vi "ShooterControl.vi"(0 "ShooterTop":T1={"DeviceStatus"={"status"=FALSE, "code"=0, "source"=""}, "Type"=enum."PWM", "PWM"={"Digital Module"=enum."Digital Module 1", "PWM Channel"=enum."Invalid", "DeadBand"={"Name"="", "maxPositivePwm"=0, "minPositivePwm"=0, "centerPwm"=0, "maxNegativePwm"=0, "minNegativePwm"=0, "angularRange"=0}}, "CAN"={"Device Number"=0, "Control Mode"=enum."Percent VBus", "Semaphore"=refnum, "Max Vout"=12.0}, "Invert"=FALSE, "TransformRef"=refnum, "InvTransformRef"=refnum}, 1 "ShooterBottom":T1={"DeviceStatus"={"status"=FALSE, "code"=0, "source"=""}, "Type"=enum."PWM", "PWM"={"Digital Module"=enum."Digital Module 1", "PWM Channel"=enum."Invalid", "DeadBand"={"Name"="", "maxPositivePwm"=0, "minPositivePwm"=0, "centerPwm"=0, "maxNegativePwm"=0, "minNegativePwm"=0, "angularRange"=0}}, "CAN"={"Device Number"=0, "Control Mode"=enum."Percent VBus", "Semaphore"=refnum, "Max Vout"=12.0}, "Invert"=FALSE, "TransformRef"=refnum, "InvTransformRef"=refnum}, 2 "ThrottleAxis":dbl, 3 "AutoTrack":bool, 4 "ClosedLoopKillSwitch":bool, 5 "ON/OFF":bool, 6 "TopEnc":dbl, 7 "OpenLoopMax":dbl, 8 "BotEnc":dbl, 9 "OpenLoopMin":dbl, 10 "button6":bool, 11 "ClosedLoopMax":dbl, 12 "Distance":dbl, 13 "ClosedLoopMin":dbl, 18 "button8":bool, 19 "button7":bool) -> (14 "ShooterTop":T1={"DeviceStatus"={"status"=FALSE, "code"=0, "source"=""}, "Type"=enum."PWM", "PWM"={"Digital Module"=enum."Digital Module 1", "PWM Channel"=enum."Invalid", "DeadBand"={"Name"="", "maxPositivePwm"=0, "minPositivePwm"=0, "centerPwm"=0, "maxNegativePwm"=0, "minNegativePwm"=0, "angularRange"=0}}, "CAN"={"Device Number"=0, "Control Mode"=enum."Percent VBus", "Semaphore"=refnum, "Max Vout"=12.0}, "Invert"=FALSE, "TransformRef"=refnum, "InvTransformRef"=refnum}, 15 "ShooterTopValue":dbl, 16 "ShooterBottom":T1={"DeviceStatus"={"status"=FALSE, "code"=0, "source"=""}, "Type"=enum."PWM", "PWM"={"Digital Module"=enum."Digital Module 1", "PWM Channel"=enum."Invalid", "DeadBand"={"Name"="", "maxPositivePwm"=0, "minPositivePwm"=0, "centerPwm"=0, "maxNegativePwm"=0, "minNegativePwm"=0, "angularRange"=0}}, "CAN"={"Device Number"=0, "Control Mode"=enum."Percent VBus", "Semaphore"=refnum, "Max Vout"=12.0}, "Invert"=FALSE, "TransformRef"=refnum, "InvTransformRef"=refnum}, 17 "ShooterBottomValue":dbl)   [LabVIEW 2011]
uses:
  <vilib>/Rock Robotics/WPI/MotorControl/WPI_MotorControlDeviceRef.ctl
  <vilib>/Rock Robotics/SystemInterfaces/Typedef/FPGA_TypedefDigitalModule.ctl
  <vilib>/Rock Robotics/SystemInterfaces/DIO/FPGA_DIOPWMChannel.ctl
  <vilib>/Rock Robotics/WPI/PWM/WPI_PWMDeadband.ctl
  <vilib>/Rock Robotics/WPI/CAN/Jaguar/SubVIs/WPI_CANJaguar_ControlMode.ctl
  <vilib>/Rock Robotics/WPI/PWM/WPI_PWMTransform_ConPane.ctl
  <vilib>/Rock Robotics/WPI/DriverStation/DriverStationLCD/WPI_DriverStationLCDLCDLine.ctl
  <vilib>/Rock Robotics/WPI/CAN/Jaguar/SubVIs/WPI_CANJaguar_SpeedReference.ctl
  Robot Global Data.vi
panel:
  in  "Add Num":dbl
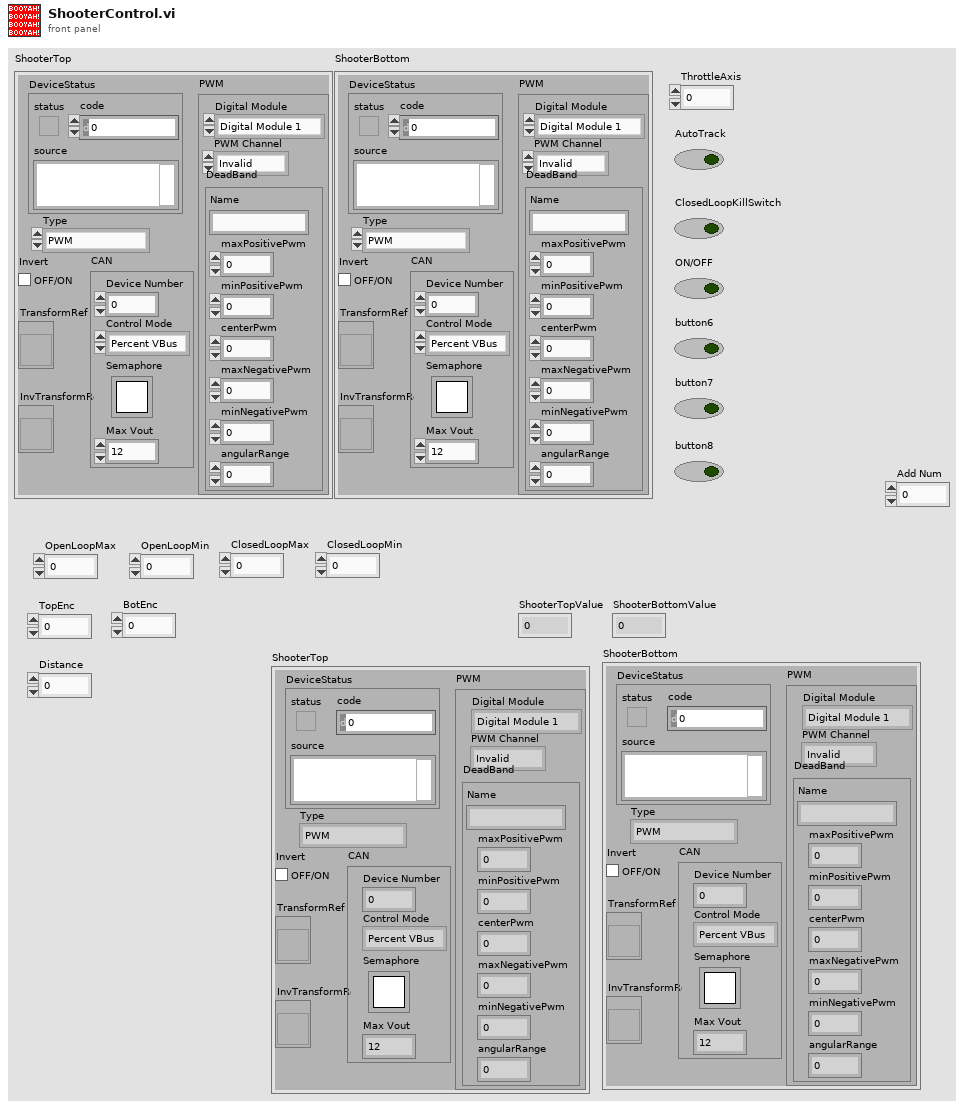
[diagram p1: front panel]
types:
  T1 = typedef "WPI_MotorControlDeviceRef.ctl" = cluster{"DeviceStatus":errorcluster, "Type":enum16{"PWM", "CAN"}, "PWM":cluster{"Digital Module":T2, "PWM Channel":T3, "DeadBand":T4}, "CAN":cluster{"Device Number":u8, "Control Mode":T5, "Semaphore":T6, "Max Vout":dbl}, "Invert":bool, "TransformRef":T7, "InvTransformRef":T7}
  T2 = typedef "FPGA_TypedefDigitalModule.ctl" = enum16{"Digital Module 1", "Digital Module 2"}
  T3 = typedef "FPGA_DIOPWMChannel.ctl" = enum8{"PWM 1", "PWM 2", "PWM 3", "PWM 4", "PWM 5", "PWM 6", "PWM 7", "PWM 8", "PWM 9", "PWM 10", "Invalid"}
  T4 = typedef "WPI_PWMDeadband.ctl" = cluster{"Name":string, "maxPositivePwm":i32, "minPositivePwm":i32, "centerPwm":i32, "maxNegativePwm":i32, "minNegativePwm":i32, "angularRange":u16}
  T5 = typedef "WPI_CANJaguar_ControlMode.ctl" = enum8{"Percent VBus", "Current", "Speed", "Position", "Voltage"}
  T6 = typedef "Semaphore RefNum" = refnum<k1>
  T7 = typedef "WPI_PWMTransform_ConPane.ctl" = refnum<vi>
  T8 = typedef "WPI_DriverStationLCDLCDLine.ctl" = enum16{"Main - Line 1", "User - Line 2", "User - Line 3", "User - Line 4", "User - Line 5", "User - Line 6"}
  T9 = typedef "WPI_CANJaguar_SpeedReference.ctl" = u8
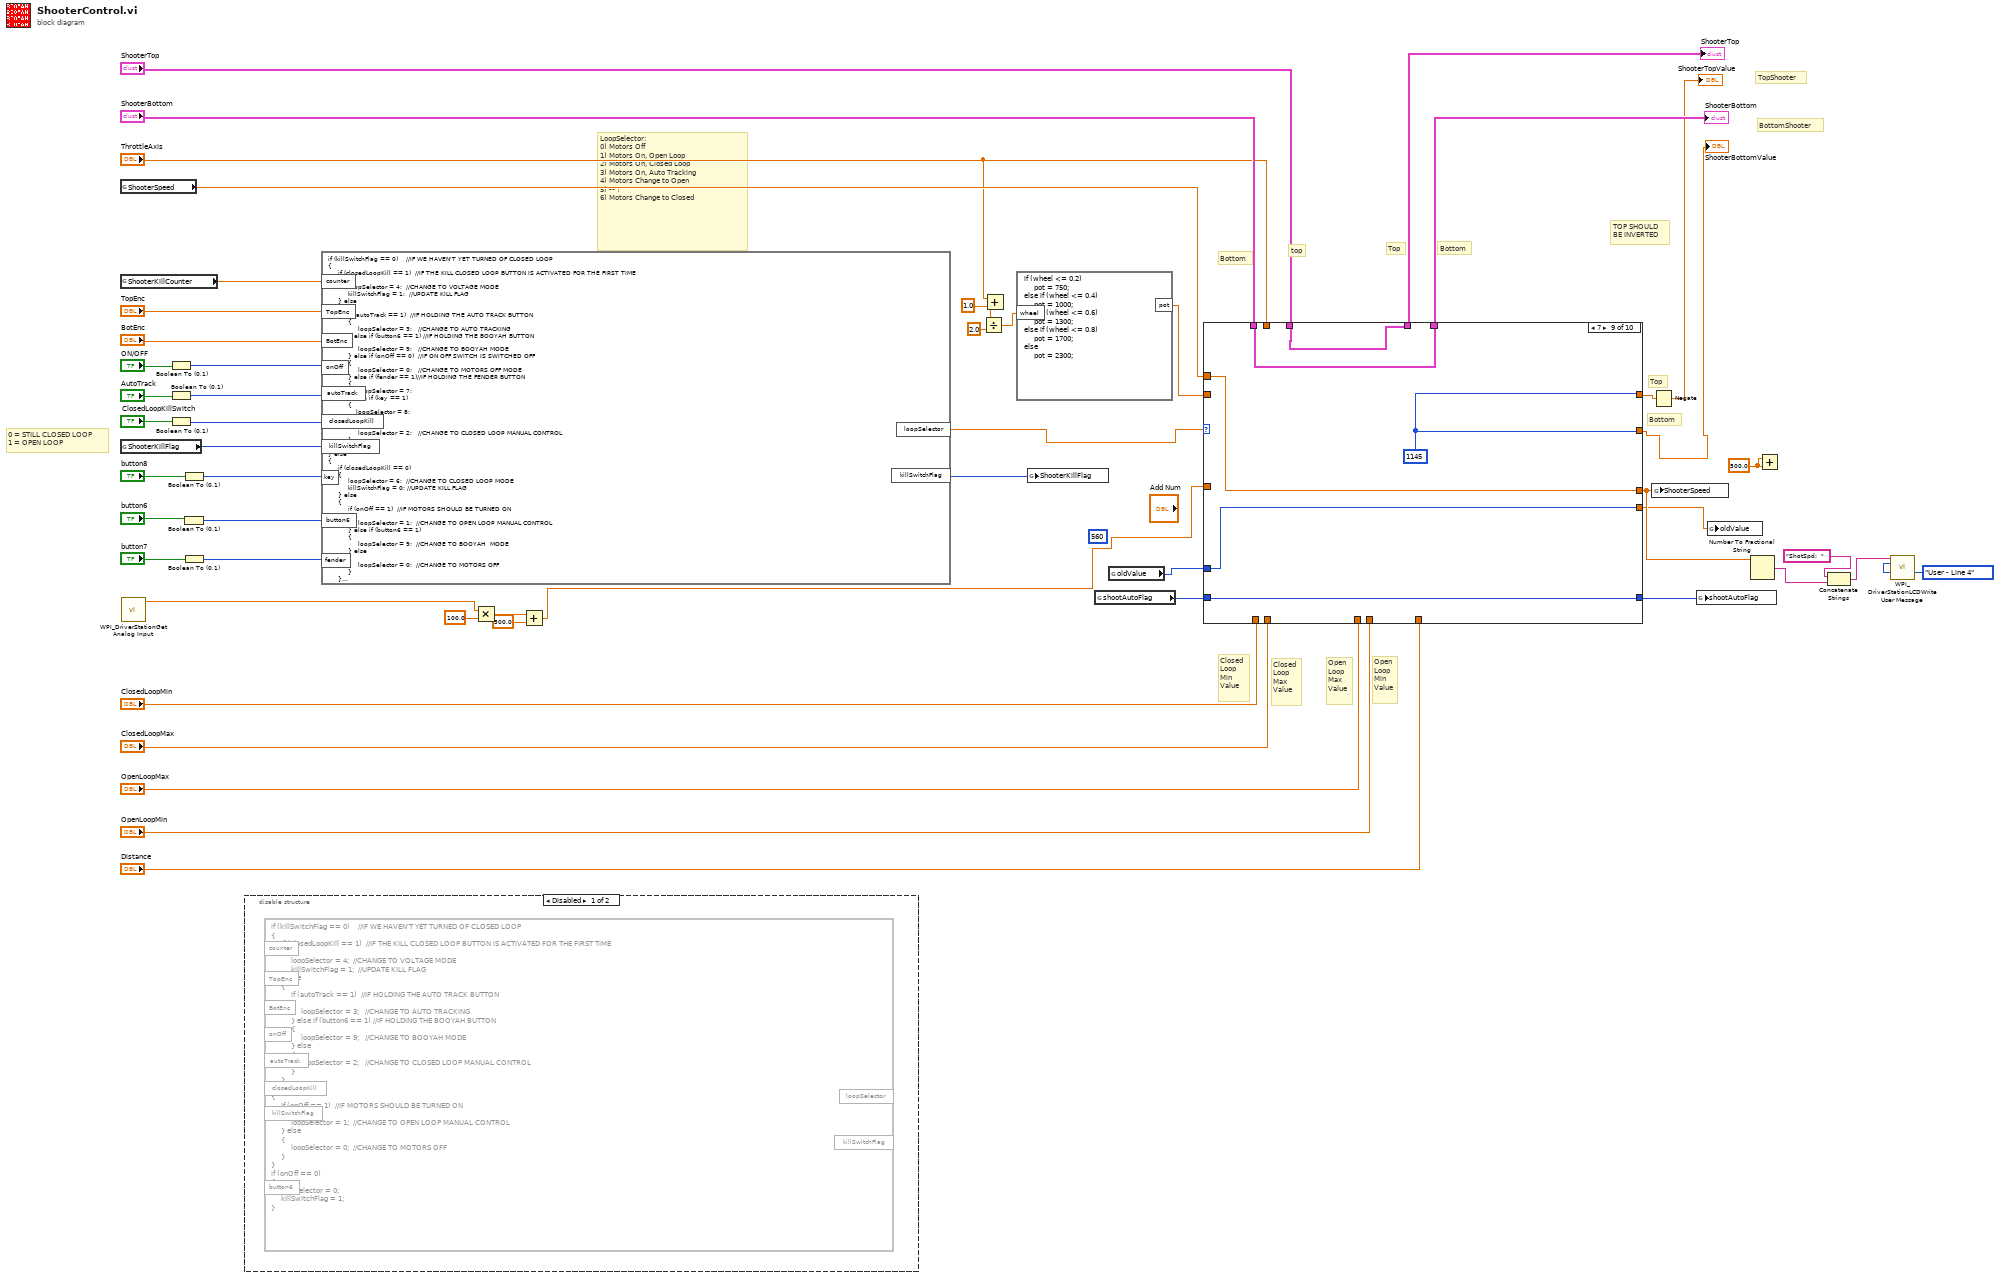
[diagram p0: block diagram]
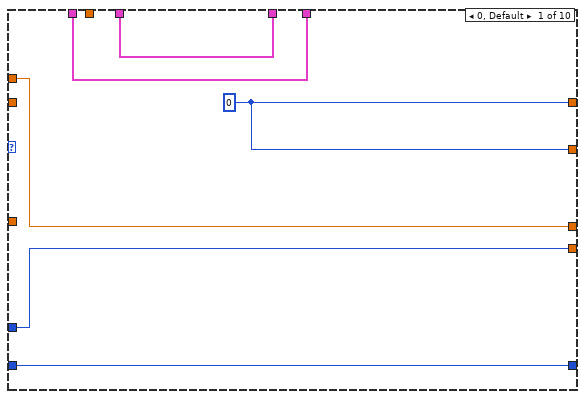
[diagram p3: hidden frame]
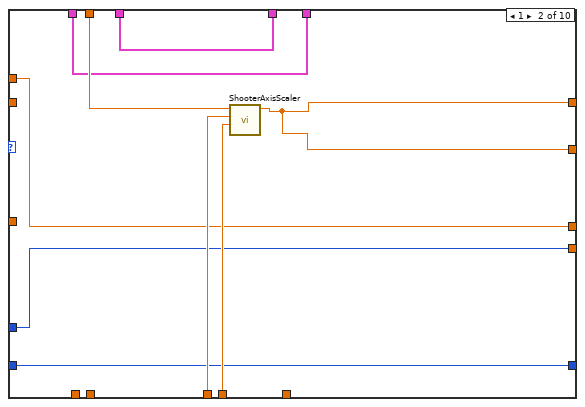
[diagram p4: hidden frame]
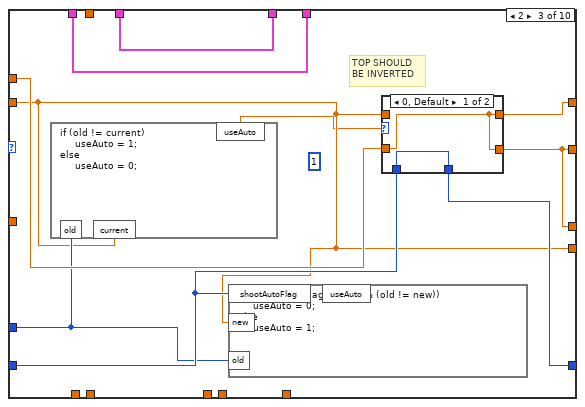
[diagram p5: hidden frame]
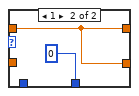
[diagram p6: hidden frame]
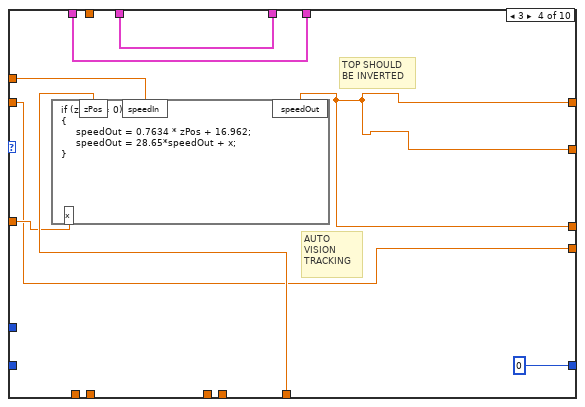
[diagram p7: hidden frame]
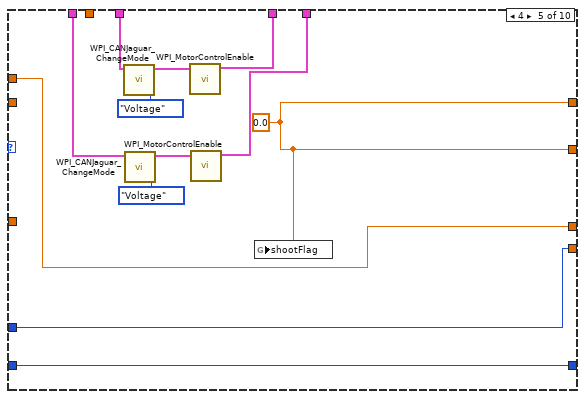
[diagram p8: hidden frame]
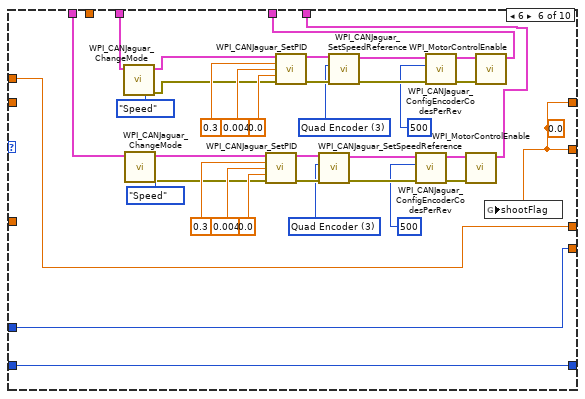
[diagram p9: hidden frame]
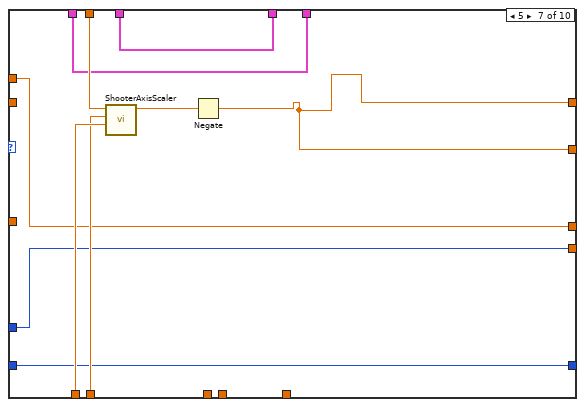
[diagram p10: hidden frame]
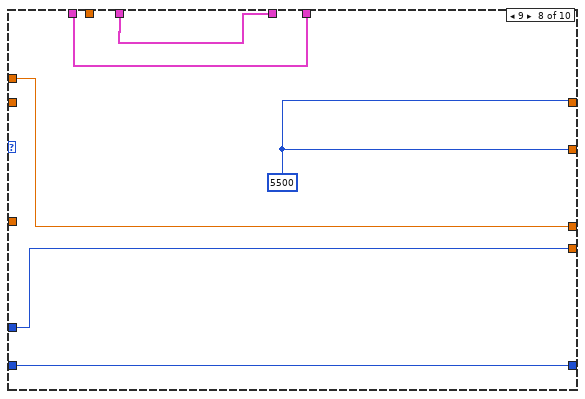
[diagram p11: hidden frame]
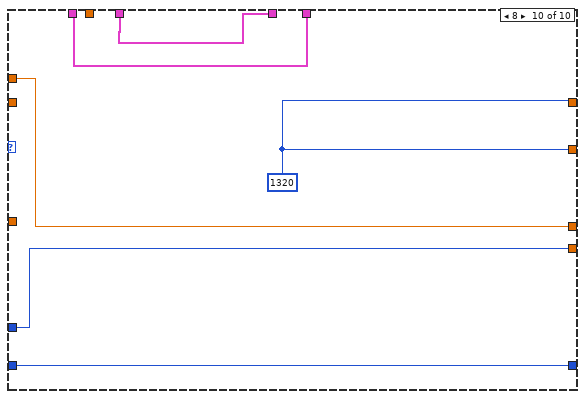
[diagram p12: hidden frame]
diagram:
  (unwired) 560
  w26 = 500.0 ("y")
  # "TOP SHOULD\nBE INVERTED"
  # "0 = STILL CLOSED LOOP\n1 = OPEN LOOP"
  # "Bottom"
  # "Top"
  # "top"
  # "Bottom"
  # "Closed\nLoop\nMin\nValue"
  # "Closed\nLoop\nMax\nValue"
  # "Open\nLoop\nMax\nValue"
  # "Open\nLoop\nMin\nValue"
  # "Bottom"
  # "BottomShooter"
  # "TopShooter"
  # "Top"
  # "LoopSelector:\n0) Motors Off\n1) Motors On, Open Loop\n2) Motors On, Closed Loop\n3) Motors On, Auto Tracking\n4) Motors Change to Open\n5) -- ?\n6) Motors Change to Closed"
  n1 = global read "Robot Global Data.vi" "ShooterSpeed"() -> (w29:dbl)
  n2 = global read "Robot Global Data.vi" "ShooterKillCounter"() -> (w33:dbl)
  n3 = global read "Robot Global Data.vi" "ShooterKillFlag"() -> (w38:u8)
  n4 = call <vilib>:"WPI_DriverStationGet Analog Input.vi"() -> ("Analog 1 (V)"=w23:dbl)  [unwired: 8 in, 3 out]
  n5 = Boolean To (0,1)(Boolean="ON/OFF") -> (0, 1=w47:i16)
  n6 = Boolean To (0,1)(Boolean="AutoTrack") -> (0, 1=w49:i16)
  n7 = Boolean To (0,1)(Boolean="ClosedLoopKillSwitch") -> (0, 1=w51:i16)
  n8 = Boolean To (0,1)(Boolean="button6") -> (0, 1=w31:i16)
  n9 = Boolean To (0,1)(Boolean="button8") -> (0, 1=w2:i16)
  n10 = Boolean To (0,1)(Boolean="button7") -> (0, 1=w24:i16)
  n11 = disable-structure shown="Disabled" {
    frame Disabled {
      n12 = formula code="if (killSwitchFlag == 0)    //IF WE HAVEN'T YET TURNED OF CLOSED LOOP\n{\n     if (closedLoopKill == 1)  //IF THE KILL CLOSED LOOP BUTTON IS ACTIVATED FOR THE FIRST TIME\n     {\n          loopSelector = 4;  //CHANGE TO VOLTAGE MODE\n          killSwitchFlag = 1;  //UPDATE KILL FLAG\n     } else\n     {\n          if (autoTrack == 1)  //IF HOLDING THE AUTO TRACK BUTTON\n          {\n               loopSelector = 3;   //CHANGE TO AUTO TRACKING\n          } else if (button6 == 1) //IF HOLDING THE BOOYAH BUTTON\n          {\n               loopSelector = 9;   //CHANGE TO BOOYAH MODE\n          } else\n          {\n               loopSelector = 2;   //CHANGE TO CLOSED LOOP MANUAL CONTROL\n          }\n     }\n} else\n{\n     if (onOff == 1)  //IF MOTORS SHOULD BE TURNED ON\n     {\n          loopSelector = 1;  //CHANGE TO OPEN LOOP MANUAL CONTROL\n     } else\n     {\n          loopSelector = 0;  //CHANGE TO MOTORS OFF\n     }\n}\nif (onOff == 0)\n{\n     loopSelector = 0;\n     killSwitchFlag = 1;\n}"() -> ()  [unwired: 8 in, 2 out]
    }
    frame Enabled {
    }
  }
  n13 = formula code="if (killSwitchFlag == 0)    //IF WE HAVEN'T YET TURNED OF CLOSED LOOP\n{\n     if (closedLoopKill == 1)  //IF THE KILL CLOSED LOOP BUTTON IS ACTIVATED FOR THE FIRST TIME\n     {\n          loopSelector = 4;  //CHANGE TO VOLTAGE MODE\n          killSwitchFlag = 1;  //UPDATE KILL FLAG\n     } else\n     {\n          if (autoTrack == 1)  //IF HOLDING THE AUTO TRACK BUTTON\n          {\n               loopSelector = 3;   //CHANGE TO AUTO TRACKING\n          } else if (button6 == 1) //IF HOLDING THE BOOYAH BUTTON\n          {\n               loopSelector = 9;   //CHANGE TO BOOYAH MODE\n          } else if (onOff == 0)  //IF ON OFF SWITCH IS SWITCHED OFF\n          {\n               loopSelector = 0;   //CHANGE TO MOTORS OFF MODE\n          } else if (fender == 1)//IF HOLDING THE FENDER BUTTON\n          {\n               loopSelector = 7;\n          } else if (key == 1)\n          {\n              loopSelector = 8;\n          } else \n          {\n               loopSelector = 2;   //CHANGE TO CLOSED LOOP MANUAL CONTROL\n          }\n     }\n} else\n{\n     if (closedLoopKill == 0)\n     {\n          loopSelector = 6;  //CHANGE TO CLOSED LOOP MODE\n          killSwitchFlag = 0; //UPDATE KILL FLAG\n     } else\n     {\n          if (onOff == 1)  //IF MOTORS SHOULD BE TURNED ON\n          {\n               loopSelector = 1;  //CHANGE TO OPEN LOOP MANUAL CONTROL\n          } else if (button6 == 1)\n          {\n               loopSelector = 9;  //CHANGE TO BOOYAH  MODE\n          } else          \n          {\n               loopSelector = 0;  //CHANGE TO MOTORS OFF\n          }\n     }\n}"("onOff"=w47, "autoTrack"=w49, "closedLoopKill"=w51, "killSwitchFlag"=w38, "TopEnc"="TopEnc", "BotEnc"="BotEnc", "counter"=w33, "button6"=w31, "fender"=w24, "key"=w2) -> ("loopSelector"=w36:dbl, "killSwitchFlag"=w37:u8)
  n14 = Multiply(x=w23, y=100.0) -> (x*y=w21:dbl)
  n15 = Add(x=w21, y=500.0) -> (x+y=w19:dbl)
  n16 = Add(x="ThrottleAxis", y=1.0) -> (x+y=w9:dbl)
  n17 = Divide(x=w9, y=2.0) -> (x/y=w11:dbl)
  n18 = formula code="if (wheel <= 0.2)\n     pot = 750;\nelse if (wheel <= 0.4)\n     pot = 1000;\nelse if (wheel <= 0.6)\n     pot = 1300;\nelse if (wheel <= 0.8)\n     pot = 1700;\nelse\n     pot = 2300;"("wheel"=w11) -> ("pot"=w6:dbl)
  n19 = global write "Robot Global Data.vi" "ShooterKillFlag"(w37) -> ()
  n20 = global read "Robot Global Data.vi" "shootAutoFlag"() -> (w27:i8)
  n21 = global read "Robot Global Data.vi" "oldValue"() -> (w12:i32)
  n22 = case shown="7" w36 {
    tunnel: [w58 w60 w75 w84 w93 w133 w139 w149 w155 w161] -> w3
    tunnel: [w58 w60 w71 w84 w93 w133 w139 w149 w155 w161] -> w5
    tunnel: "OpenLoopMax" -> [_ w67 _ _ _ _ _ _ _ _]
    tunnel: "OpenLoopMin" -> [_ w66 _ _ _ _ _ _ _ _]
    tunnel: "ThrottleAxis" -> [_ w65 _ _ _ _ w147 _ _ _]
    tunnel: "ClosedLoopMin" -> [_ _ _ _ _ _ w146 _ _ _]
    tunnel: "ClosedLoopMax" -> [_ _ _ _ _ _ w145 _ _ _]
    tunnel: "ShooterTop" -> [w57 w64 w77 w89 w97 w135 w144 w153 w159 w165]
    tunnel: "ShooterBottom" -> [w56 w63 w76 w88 w96 w134 w143 w152 w158 w164]
    tunnel: [w57 w64 w77 w89 w95 w105 w144 w153 w159 w165] -> w40
    tunnel: [w56 w63 w76 w88 w94 w104 w143 w152 w158 w164] -> w39
    tunnel: "Distance" -> [_ _ _ w87 _ _ _ _ _ _]
    tunnel: [w55 w62 w71 w84 w92 w132 w141 w151 w157 w163] -> w14
    tunnel: w29 -> [w55 w62 w72 w86 w92 w132 w141 w151 w157 w163]
    tunnel: [w54 w61 w74 0 w91 w103 w140 w150 w156 w162] -> w28
    tunnel: w27 -> [w54 w61 w73 _ w91 w103 w140 w150 w156 w162]
    tunnel: [w53 w59 w69 w82 w90 w102 w138 w148 w154 w160] -> w13
    tunnel: w12 -> [w53 w59 w70 _ w90 w102 w138 w148 w154 w160]
    tunnel: w19 -> [_ _ _ w83 _ _ _ _ _ _]
    tunnel: w6 -> [_ _ w69 w82 _ _ _ _ _ _]
    frame 0, Default {
      w58 = 0
    }
    frame 1 {
      n23 = call "ShooterAxisScaler.vi"("MinValue"=w66, "MaxValue"=w67, "ThrottleAxisIn"=w65) -> ("ScaledThrottleOut"=w60:dbl)  [unwired: 8 in]
    }
    frame 2 {
      (unwired) 1
      # "TOP SHOULD\nBE INVERTED"
      n24 = formula code="if (old != current)\n     useAuto = 1;\nelse\n     useAuto = 0;"("old"=w70, "current"=w69) -> ("useAuto"=w68:dbl)
      n25 = formula code="if ((shootAutoFlag == 1) && (old != new))\n     useAuto = 0;\nelse\n     useAuto = 1;"("shootAutoFlag"=w73, "old"=w70, "new"=w69) -> ()  [unwired: 1 out]
      n26 = case shown="0, Default" w68 {
        tunnel: [w78 w81] -> w75
        tunnel: w69 -> [_ w81]
        tunnel: [w78 w81] -> w71
        tunnel: [w79 0] -> w74
        tunnel: w73 -> [w79 _]
        tunnel: w72 -> [w78 _]
        frame 0, Default {
        }
        frame 1 {
        }
      }
    }
    frame 3 {
      # "TOP SHOULD\nBE INVERTED"
      # "AUTO\nVISION\nTRACKING"
      n27 = formula code="if (zPos != 0)\n{\n     speedOut = 0.7634 * zPos + 16.962;\n     speedOut = 28.65*speedOut + x;\n}"("zPos"=w87, "speedIn"=w86, "x"=w83) -> ("speedOut"=w84:dbl)
    }
    frame 4 {
      w93 = 0.0 ("ScaledThrottleOut")
      n28 = call <vilib>:"WPI_CANJaguar_ChangeMode.vi"("Control Mode"=WPI_CANJaguar_ControlMode."Voltage", "CAN Jaguar Ref"=w97) -> ("CAN Jaguar Ref Out"=w100:T1)  [unwired: 1 in, 8 out]
      n29 = call <vilib>:"WPI_CANJaguar_ChangeMode.vi"("Control Mode"=WPI_CANJaguar_ControlMode."Voltage", "CAN Jaguar Ref"=w96) -> ("CAN Jaguar Ref Out"=w98:T1)  [unwired: 1 in, 8 out]
      n30 = call <vilib>:"WPI_MotorControlEnable.vi"("CAN Jaguar Ref"=w100) -> ("CAN Jaguar Ref Out"=w95:T1)  [unwired: 2 in, 8 out]
      n31 = call <vilib>:"WPI_MotorControlEnable.vi"("CAN Jaguar Ref"=w98) -> ("CAN Jaguar Ref Out"=w94:T1)  [unwired: 2 in, 8 out]
      n32 = global write "Robot Global Data.vi" "shootFlag"(w93) -> ()
    }
    frame 6 {
      w113 = T9 3 items=["Encoder"=0, "Inv Encoder"=2, "Quad Encoder"=3, "None"=255] ("Speed Reference")
      w126 = T9 3 items=["Encoder"=0, "Inv Encoder"=2, "Quad Encoder"=3, "None"=255] ("Speed Reference")
      w133 = 0.0 ("ScaledThrottleOut")
      n33 = call <vilib>:"WPI_CANJaguar_ChangeMode.vi"("Control Mode"=WPI_CANJaguar_ControlMode."Speed", "CAN Jaguar Ref"=w135) -> ("error out"=w119:errorcluster, "CAN Jaguar Ref Out"=w120:T1)  [unwired: 1 in, 7 out]
      n34 = call <vilib>:"WPI_CANJaguar_ChangeMode.vi"("Control Mode"=WPI_CANJaguar_ControlMode."Speed", "CAN Jaguar Ref"=w134) -> ("error out"=w106:errorcluster, "CAN Jaguar Ref Out"=w107:T1)  [unwired: 1 in, 7 out]
      n35 = call <vilib>:"WPI_CANJaguar_SetPID.vi"("CAN Jaguar Ref"=w107, "P"=0.3, "I"=0.004, "D"=0.0, "error in (no error)"=w106) -> ("CAN Jaguar Ref Out"=w114:T1, "error out"=w115:errorcluster)  [unwired: 9 in]
      n36 = call <vilib>:"WPI_CANJaguar_SetPID.vi"("CAN Jaguar Ref"=w120, "P"=0.3, "I"=0.004, "D"=0.0, "error in (no error)"=w119) -> ("CAN Jaguar Ref Out"=w127:T1, "error out"=w128:errorcluster)  [unwired: 9 in]
      n37 = call <vilib>:"WPI_CANJaguar_SetSpeedReference.vi"("error in (no error)"=w115, "Speed Reference"=w113, "CAN Jaguar Ref"=w114) -> ("error out"=w112:errorcluster, "CAN Jaguar Ref Out"=w111:T1)  [unwired: 7 in]
      n38 = call <vilib>:"WPI_CANJaguar_SetSpeedReference.vi"("error in (no error)"=w128, "Speed Reference"=w126, "CAN Jaguar Ref"=w127) -> ("error out"=w125:errorcluster, "CAN Jaguar Ref Out"=w124:T1)  [unwired: 7 in]
      n39 = call <vilib>:"WPI_CANJaguar_ConfigEncoderCodesPerRev.vi"("error in (no error)"=w112, "Encoder Codes Per Rev"=u16 500, "CAN Jaguar Ref"=w111) -> ("error out"=w108:errorcluster, "CAN Jaguar Ref Out"=w109:T1)  [unwired: 7 in]
      n40 = call <vilib>:"WPI_CANJaguar_ConfigEncoderCodesPerRev.vi"("error in (no error)"=w125, "Encoder Codes Per Rev"=u16 500, "CAN Jaguar Ref"=w124) -> ("error out"=w121:errorcluster, "CAN Jaguar Ref Out"=w122:T1)  [unwired: 7 in]
      n41 = call <vilib>:"WPI_MotorControlEnable.vi"("error in (no error)"=w108, "CAN Jaguar Ref"=w109) -> ("CAN Jaguar Ref Out"=w104:T1)  [unwired: 8 in, 1 out]
      n42 = call <vilib>:"WPI_MotorControlEnable.vi"("error in (no error)"=w121, "CAN Jaguar Ref"=w122) -> ("CAN Jaguar Ref Out"=w105:T1)  [unwired: 8 in, 1 out]
      n43 = global write "Robot Global Data.vi" "shootFlag"(w133) -> ()
    }
    frame 5 {
      n44 = call "ShooterAxisScaler.vi"("MinValue"=w146, "MaxValue"=w145, "ThrottleAxisIn"=w147) -> ("ScaledThrottleOut"=w142:dbl)  [unwired: 8 in]
      n45 = Negate(x=w142) -> (-x=w139:dbl)
    }
    frame 9 {
      w149 = 5500
    }
    frame 7 {
      w155 = 1145
    }
    frame 8 {
      w161 = 1320
    }
  }
  "ShooterTop" <- w40
  "ShooterBottom" <- w39
  "ShooterBottomValue" <- w5
  n46 = Negate(x=w3) -> (-x=→"ShooterTopValue":dbl)
  n47 = global write "Robot Global Data.vi" "ShooterSpeed"(w14) -> ()
  n48 = global write "Robot Global Data.vi" "shootAutoFlag"(w28) -> ()
  n49 = global write "Robot Global Data.vi" "oldValue"(w13) -> ()
  n50 = Number To Fractional String(number=w14) -> (F-format string=w16:string)  [unwired: 3 in]
  n51 = Add(x=w26, y=w26) -> ()  [unwired: 1 out]
  n52 = Concatenate Strings("ShotSpd:  " ("line text"), w16) -> (w15:string)
  n53 = call <vilib>:"WPI_DriverStationLCDWrite User Message.vi"("line text"=w15, "line"=WPI_DriverStationLCDLCDLine."User - Line 4") -> ()  [unwired: 13 in, 1 out]
